vi "VITester_Item_NotifyChanged.vi"(8 "error in":errorcluster, 10 "Change Type":T1=enum."Item Modified", 11 "Object":T2) -> (0 "error out":errorcluster)   [LabVIEW 2013]
uses:
  <resource>/Framework/Providers/vitester-src/Support/VITester Project Item Ref.ctl
  <resource>/Framework/Providers/API/mxLvChangeType.ctl
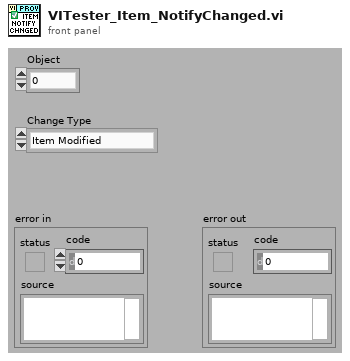
[diagram p1: front panel]
types:
  T1 = typedef "mxLvChangeType.ctl" = enum32{"Item Created", "Item Modified", "File Modified", "File Deleted", "Item Added", "Item Added to SCC", "Item Renamed", "Item Modified For SCC"}
  T2 = typedef "VITester Project Item Ref.ctl" = u64
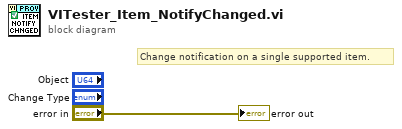
[diagram p0: block diagram]
diagram:
  # "Change notification on a single supported item."
  "error out" <- "error in"
